vi "String Equals.vi"(8 "error in (no error)":errorcluster, 10 "Data DVR in":refnum<data-value>, 11 "String DVR in":refnum<data-value>) -> (0 "error out":errorcluster, 1 "Equals?":bool, 2 "Data DVR out":refnum<data-value>, 3 "String DVR out":refnum<data-value>)   [LabVIEW 2012, in "MDSplus.lvlib"]
doc: "Write data for this node."
uses:
  <vilib>/MDSplus/Library/MDSplus.lvlib
  <vilib>/MDSplus/Classes/Data_Class/Scalar_Class/String_Class/String.lvclass
  <vilib>/MDSplus/Classes/Data_Class/Data.lvclass
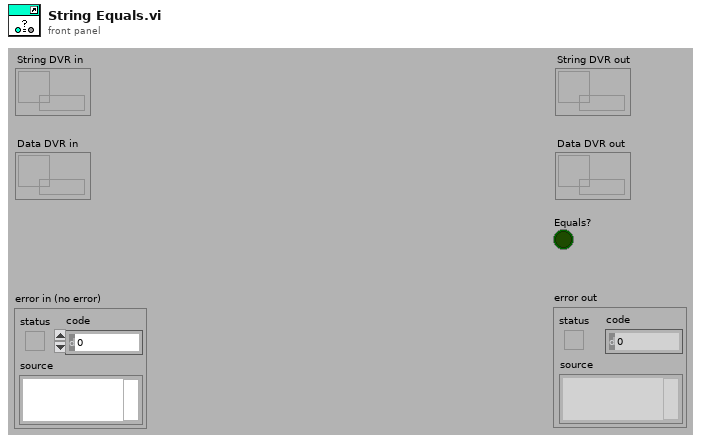
[diagram p1: front panel]
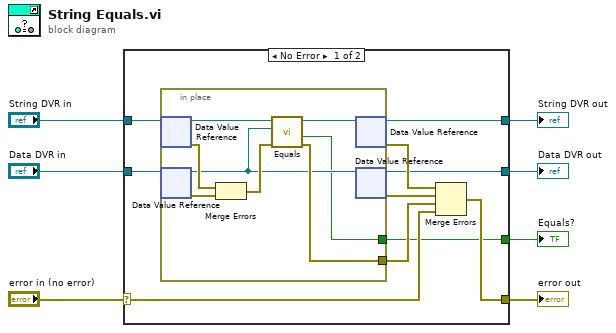
[diagram p0: block diagram]
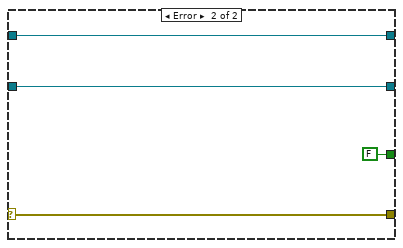
[diagram p2: hidden frame]
diagram:
  n1 = case shown="No Error" "error in (no error)" {
    selector: "error in (no error)" -> [w11 w27]
    tunnel: "String DVR in" -> [w17 w29]
    tunnel: [w14 w27] -> w7
    tunnel: [w15 w29] -> w4
    tunnel: "Data DVR in" -> [w13 w28]
    tunnel: [w9 w28] -> w2
    tunnel: [w8 FALSE ("Equals?")] -> w1
    frame No Error {
      n2 = in-place {
        in-place-border: [w20] -> w10
        in-place-border: [w18] -> w8
        n3 = in-place-dvr #1(w17) -> (w25:refnum<class "String.lvclass">, w23:errorcluster)
        n4 = in-place-dvr #2(w13) -> (w19:refnum<class "Data.lvclass">, w22:errorcluster)
        n5 = Merge Errors(w23, w22) -> (w21:errorcluster)
        n6 = call-dynamic "Equals.vi"("error in (no error)"=w21, "Data in"=w19, "String in"=w25) -> ("error out"=w20:errorcluster, "Equals?"=w18:bool, "String out"=w24:refnum<class "String.lvclass">)  [unwired: 5 in, 1 out]
        n7 = in-place-dvr #1(w24) -> (w15:refnum<data-value>, w16:errorcluster)
        n8 = in-place-dvr #2(w19) -> (w9:refnum<data-value>, w12:errorcluster)
      }
      n9 = Merge Errors(w16, w12, w10, w11) -> (w14:errorcluster)
    }
    frame Error {
    }
  }
  "error out" <- w7
  "String DVR out" <- w4
  "Data DVR out" <- w2
  "Equals?" <- w1
